vi "Resolve Relative URI.vi"(7 "Base URI":refnum<class "URI.lvclass">, 10 "error in (no error)":errorcluster, 11 "URI in":refnum<class "URI.lvclass">) -> (2 "error out":errorcluster, 3 "URI out":refnum<class "URI.lvclass">)   [LabVIEW 2020, in "URI.lvlib" / "URI.lvclass"]
uses:
  URI.lvclass
  URI.lvclass/URI.ctl
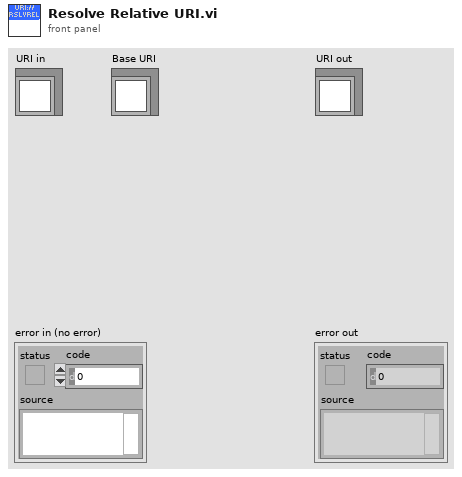
[diagram p1: front panel]
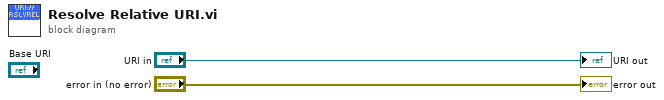
[diagram p0: block diagram]
diagram:
  "error out" <- "error in (no error)"
  "URI out" <- "URI in"
